vi "Engine.vi"(8 "error in (no error)":errorcluster) -> (0 "error out":errorcluster, 3 "Engine":refnum<class "Engine.lvclass">)   [LabVIEW 2024, in "GLF.lvlib" / "Engine.lvclass"]
uses:
  Engine.lvclass
  Engine.lvclass/Engine.ctl
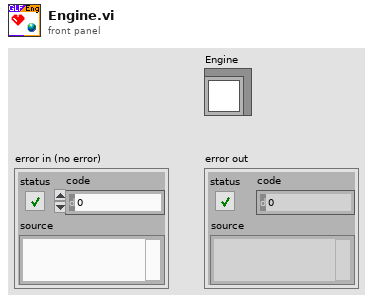
[diagram p1: front panel]
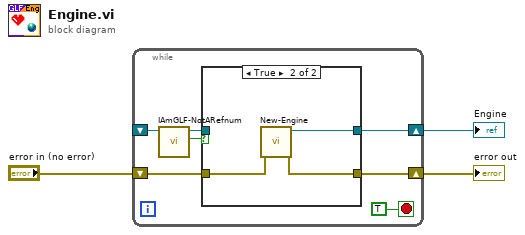
[diagram p0: block diagram]
diagram:
  n1 = while {
    shift-right: [w9] -> w1
    shift-left: _ -> [w6]
    shift-right: [w7] -> w2
    shift-left: "error in (no error)" -> [w8]
    stop <- TRUE stop-if-true
    n2 = call-dynamic "IAmGLF-NotARefnum.vi"("Engine in"=w6) -> ("Not A Valid Refnum?"=w4:bool, "Engine out"=w5:refnum<class "Engine.lvclass">)  [unwired: 9 in]
    n3 = case shown="True" w4 {
      tunnel: [w12 w15] -> w9
      tunnel: w8 -> [w11 w14]
      tunnel: [w11 w13] -> w7
      tunnel: w5 -> [w12 _]
      frame False {
      }
      frame True {
        n4 = call "New-Engine.vi"("error in (no error)"=w14) -> ("error out"=w13:errorcluster, "Engine"=w15:refnum<class "Engine.lvclass">)  [unwired: 9 in]
      }
    }
  }
  "error out" <- w2
  "Engine" <- w1
